vi "TaskMon_MemoryMonitor.vi"(7 "SynchronizationRefs":T2, 8 "error in (no error)":errorcluster, 11 "VI Server Cluster":T1={"Refs"=[], "Labels"=["Label", "Size", "Font", "Heght", "Width", "Ledding Denominator", "Ledding Nominator", "Label Number", "Microstep Resolution", "X", "Y", "Z", "Italic?", "Underlined?"], "VI Ref"=refnum}) -> (0 "error out":errorcluster)   [LabVIEW 2020]
uses:
  toolkits_lv2013_32bit/VI Server ToolKit/VIS_Libraries/VI Server_Get Controls.llb/Recover M-Column ListBox.vi
  toolkits_lv2013_32bit/VI Server ToolKit/VIS_Libraries/VI Server_Get Controls.llb/Recover Text Ring DBL.vi
  Synchronization.llb/TaskMon_SynchronizationRef.ctl
  toolkits_lv2013_32bit/VI Server ToolKit/Labels&Control References.ctl
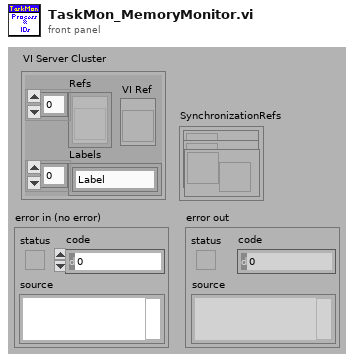
[diagram p1: front panel]
types:
  T1 = typedef "Labels&Control References.ctl" = cluster{"Refs":refnum<vi>[], "Labels":string[], "VI Ref":refnum<vi>}
  T2 = typedef "TaskMon_SynchronizationRef.ctl" = cluster{"STOP":refnum<notifier>, "PID":refnum<notifier>, "Process":refnum<notifier>}
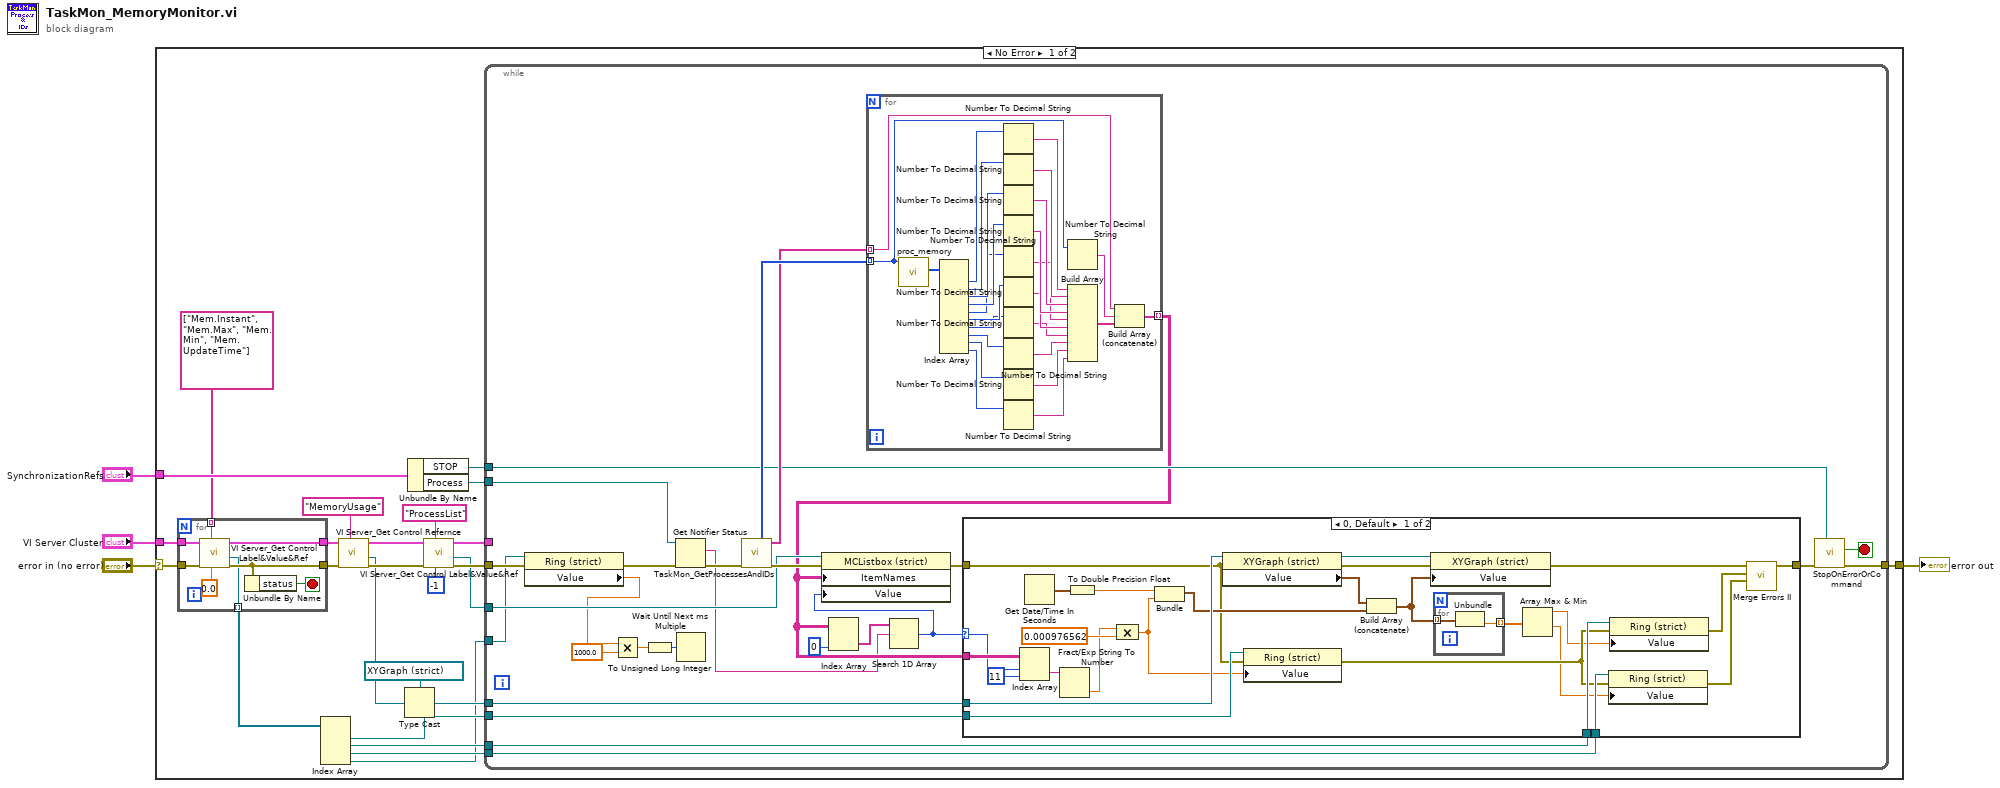
[diagram p0: block diagram]
diagram:
  n1 = case shown="No Error" "error in (no error)" {
    selector: "error in (no error)" -> [w14 w121]
    tunnel: "VI Server Cluster" -> [w16 _]
    tunnel: "SynchronizationRefs" -> [w25 _]
    tunnel: [w23 w121] -> w2
    frame No Error {
      n2 = for {
        tunnel: w16 -> [w37]
        tunnel: [w36] -> w15
        tunnel: w14 -> [w35]
        tunnel: [w33] -> w13
        tunnel: string[] ["Mem.Instant", "Mem.Max", "Mem.Min", "Mem.UpdateTime"] -> [w31] mode=indexing
        tunnel: [w30] -> w11 mode=indexing
        stop <- w32 stop-if-true
        n3 = call-poly "VI Server_Get Control Label&Value&Ref.vi"("Default Value"=0.0 ("Mem.Instant 2"), "Label"=w31, "error in"=w35, "Data Cluster"=w37) -> ("error out"=w33:errorcluster, "Control Ref"=w30:refnum<vi>, "Data Cluster dup"=w36:T1)  [unwired: 3 in, 2 out]
        n4 = Unbundle By Name(w33) -> ("status"=w32:bool)
      }
      n5 = Index Array(array=w11) -> (element #1=w10:refnum<vi>, element #2=w9:refnum<vi>, element #3=w8:refnum<vi>, element #4=w5:refnum<vi>)  [unwired: 4 in]
      n6 = call "VI Server_Get Control Refernce.vi"("Label"="MemoryUsage", "error in"=w13, "VI Server Cluster"=w15) -> ("error out"=w21:errorcluster, "Control Reference"=w19:refnum<vi>, "VI Server Cluster DUP"=w22:T1)  [unwired: 5 in, 1 out]
      n7 = Type Cast(type=refnum<vi> refnum ("MemoryUsage"), x=w19) -> (*(type *) &x=w17:refnum<vi>)
      n8 = Unbundle By Name(w25) -> ("STOP"=w24:refnum<notifier>, "Process"=w6:refnum<notifier>)
      n9 = call-poly "VI Server_Get Control Label&Value&Ref.vi"("Default Value"=-1 ("ProcessList"), "Label"="ProcessList", "error in"=w21, "Data Cluster"=w22) -> ("error out"=w29:errorcluster, "M-CLMN LIST BOX REF"=w26:refnum<vi>, "Data Cluster dup"=w7:T1)  [unwired: 3 in, 2 out]
      n10 = while {
        tunnel: w29 -> [w44]
        tunnel: w26 -> [w61]
        tunnel: w24 -> [w60]
        tunnel: [w59] -> w23
        tunnel: w17 -> [w57]
        tunnel: w10 -> [w56]
        tunnel: w9 -> [w55]
        tunnel: w8 -> [w54]
        tunnel: w7 -> [_]
        tunnel: w6 -> [w51]
        tunnel: w5 -> [w42]
        stop <- w58 stop-if-true
        n11 = property class="Ring (strict)"(reference=w42, error in=w44) -> (error out=w43:errorcluster, "Value"=w39:dbl)  [unwired: 1 out]
        n12 = Multiply(x=w39, y=1000.0) -> (x*y=w38:dbl)
        n13 = To Unsigned Long Integer(number=w38) -> (unsigned 32bit integer=w41:u32)
        n14 = Get Notifier Status(notifier=w51, error in (no error)=w43) -> (current notification=w46:string, error out=w52:errorcluster)  [unwired: 3 out]
        n15 = Wait Until Next ms Multiple(millisecond multiple=w41) -> ()  [unwired: 1 out]
        n16 = call "TaskMon_GetProcessesAndIDs.vi"("error in (no error)"=w52) -> ("error out"=w62:errorcluster, "ProcesesList"=w63:string[], "IDs"=w64:u32[])  [unwired: 2 in, 6 out]
        n17 = for {
          tunnel: w64 -> [w111] mode=indexing
          tunnel: w63 -> [w110] mode=indexing
          tunnel: [w107] -> w49 mode=indexing
          n18 = call "proc_memory.vi"("id"=w111) -> ("info 2"=w106:u32[])  [unwired: 10 out]
          n19 = Index Array(array=w106) -> (element #1=w105:u32, element #2=w104:u32, element #3=w103:u32, element #4=w102:u32, element #5=w101:u32, element #6=w100:u32, element #7=w99:u32, element #8=w98:u32, element #9=w97:u32, element #10=w96:u32)  [unwired: 10 in]
          n20 = Number To Decimal String(number=w105) -> (decimal integer string=w120:string)  [unwired: 1 out]
          n21 = Number To Decimal String(number=w104) -> (decimal integer string=w119:string)  [unwired: 1 out]
          n22 = Number To Decimal String(number=w103) -> (decimal integer string=w118:string)  [unwired: 1 out]
          n23 = Number To Decimal String(number=w102) -> (decimal integer string=w117:string)  [unwired: 1 out]
          n24 = Number To Decimal String(number=w101) -> (decimal integer string=w116:string)  [unwired: 1 out]
          n25 = Number To Decimal String(number=w100) -> (decimal integer string=w115:string)  [unwired: 1 out]
          n26 = Number To Decimal String(number=w99) -> (decimal integer string=w114:string)  [unwired: 1 out]
          n27 = Number To Decimal String(number=w98) -> (decimal integer string=w113:string)  [unwired: 1 out]
          n28 = Number To Decimal String(number=w97) -> (decimal integer string=w112:string)  [unwired: 1 out]
          n29 = Number To Decimal String(number=w96) -> (decimal integer string=w95:string)  [unwired: 1 out]
          n30 = Number To Decimal String(number=w111) -> (decimal integer string=w109:string)  [unwired: 1 out]
          n31 = Build Array(w120, w119, w118, w117, w116, w115, w114, w113, w112, w95) -> (w108:string[])
          n32 = Build Array (concatenate)(w110, w109, w108) -> (w107:string[])
        }
        n33 = Index Array(array=w49, index (col)=0 ("disabled index (col)")) -> (element=w48:string[])  [unwired: 1 in]
        n34 = Search 1D Array(1D array=w48, element=w46) -> (index of element=w45:i32)  [unwired: 1 in]
        n35 = property on="Property Node" class="MCListbox (strict)"(reference=w61, error in=w62, "ItemNames"=w49, "Value"=w45) -> (error out=w50:errorcluster)  [unwired: 1 out]
        n36 = case shown="0, Default" w45 {
          selector: w45 -> [w65 _]
          tunnel: w49 -> [w91 _]
          tunnel: w57 -> [w90 _]
          tunnel: w56 -> [w89 _]
          tunnel: w55 -> [w88 _]
          tunnel: w54 -> [w87 _]
          tunnel: [w86 w94] -> w53
          tunnel: w50 -> [w75 w94]
          frame 0, Default {
            n37 = Index Array(array=w91, index (row)=w65, index (col)=11 ("disabled index (col)")) -> (element=w83:string)
            n38 = Get Date/Time In Seconds() -> (seconds since 1Jan1904=w81:timestamp)
            n39 = Fract/Exp String To Number(string=w83) -> (number=w84:dbl)  [unwired: 3 in, 1 out]
            n40 = To Double Precision Float(number=w81) -> (double precision float=w80:dbl)
            n41 = Compound Arithmetic op=MULTIPLY(w84, 0.000976562 ("value")) -> (w74:dbl)
            n42 = Bundle(w80, w74) -> (w77:cluster{dbl, dbl})  [unwired: 1 in]
            n43 = property class="XYGraph (strict)"(reference=w90, error in=w75) -> (reference out=w76:refnum<vi>, error out=w79:errorcluster, "Value"=w78:cluster{dbl, dbl}[])
            n44 = property class="Ring (strict)"(reference=w89, error in=w75, "Value"=w74) -> (error out=w71:errorcluster)  [unwired: 1 out]
            n45 = Build Array (concatenate)(w78, w77) -> (w73:cluster{dbl, dbl}[])
            n46 = property class="XYGraph (strict)"(reference=w76, error in=w79, "Value"=w73) -> (error out=w68:errorcluster)  [unwired: 1 out]
            n47 = for {
              tunnel: w73 -> [w93] mode=indexing
              tunnel: [w92] -> w72 mode=indexing
              n48 = Unbundle(w93) -> (w92:dbl)  [unwired: 1 out]
            }
            n49 = Array Max & Min(array=w72) -> (max value=w70:dbl, min value=w69:dbl)  [unwired: 2 out]
            n50 = property class="Ring (strict)"(reference=w87, error in=w71, "Value"=w69) -> (error out=w66:errorcluster)  [unwired: 1 out]
            n51 = property class="Ring (strict)"(reference=w88, error in=w71, "Value"=w70) -> (error out=w67:errorcluster)  [unwired: 1 out]
            n52 = call "Merge Errors II.vi"("error in 3 (no error)"=w66, "error in 2 (no error)"=w67, "error in 1 (no error)"=w68) -> ("error out.DUP"=w86:errorcluster)  [unwired: 3 in, 1 out]
          }
          frame -1 {
          }
        }
        n53 = call "StopOnErrorOrCommand.vi"("STOP"=w60, "error in (no error)"=w53) -> ("error out"=w59:errorcluster, "STOP"=w58:bool)  [unwired: 8 in]
      }
    }
    frame Error {
    }
  }
  "error out" <- w2
